vi "ILABs_SetBounds.vi"(0 "viname":string, 1 "left":i16, 2 "top":i16, 3 "right":i16, 4 "appRef":refnum<vi>, 6 "bottom":i16) -> (5 "error out":errorcluster)   [LabVIEW 2009]
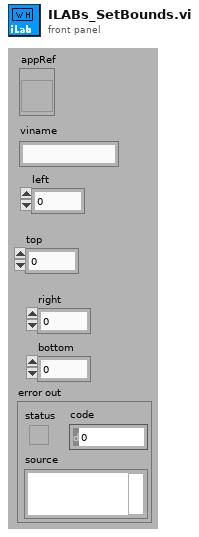
[diagram p1: front panel]
types:
  T1 = cluster{"left":i16, "top":i16, "right":i16, "bottom":i16}
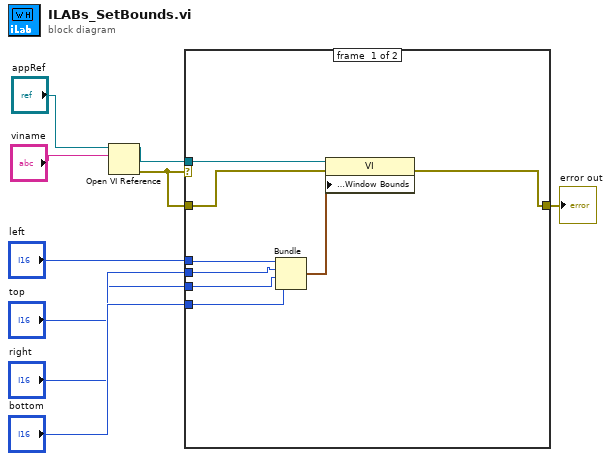
[diagram p0: block diagram]
diagram:
  n1 = Open VI Reference(application reference (local)="appRef", vi path="viname") -> (vi reference=w5:refnum<vi>, error out=w3:errorcluster)  [unwired: 1 in, 3 out]
  n2 = case shown="No Error" w3 {
    tunnel: "left" -> [w17 _]
    tunnel: "bottom" -> [w14 _]
    tunnel: "top" -> [w16 _]
    tunnel: "right" -> [w15 _]
    tunnel: w5 -> [w13 _]
    tunnel: w3 -> [w11 w18]
    tunnel: [w10 w18] -> w2
    frame #0 {
      n3 = Bundle("left"=w17, "top"=w16, "right"=w15, "bottom"=w14) -> (w12:T1)  [unwired: 1 out]
      n4 = property class="VI"(reference=w13, error in=w11, "Front Panel Window:Window Bounds"=w12) -> (error out=w10:errorcluster)  [unwired: 1 out]
    }
    frame #1 {
    }
  }
  "error out" <- w2
